vi "LabVIEW Measurement UI - Verify Parameter Matching.vi"(0 "Measurement Client Wrapper in":refnum<class "Measurement Client Wrapper.lvclass">, 11 "error in":errorcluster) -> (4 "Measurement Client Wrapper":refnum<class "Measurement Client Wrapper.lvclass">, 6 "Status":string, 8 "Matching?":bool, 15 "error out":errorcluster)   [LabVIEW 2020, in "Measurement Client Wrapper.lvclass"]
uses:
  Measurement Client Wrapper.lvclass
  Measurement Client Wrapper.lvclass/Measurement Client Wrapper.ctl
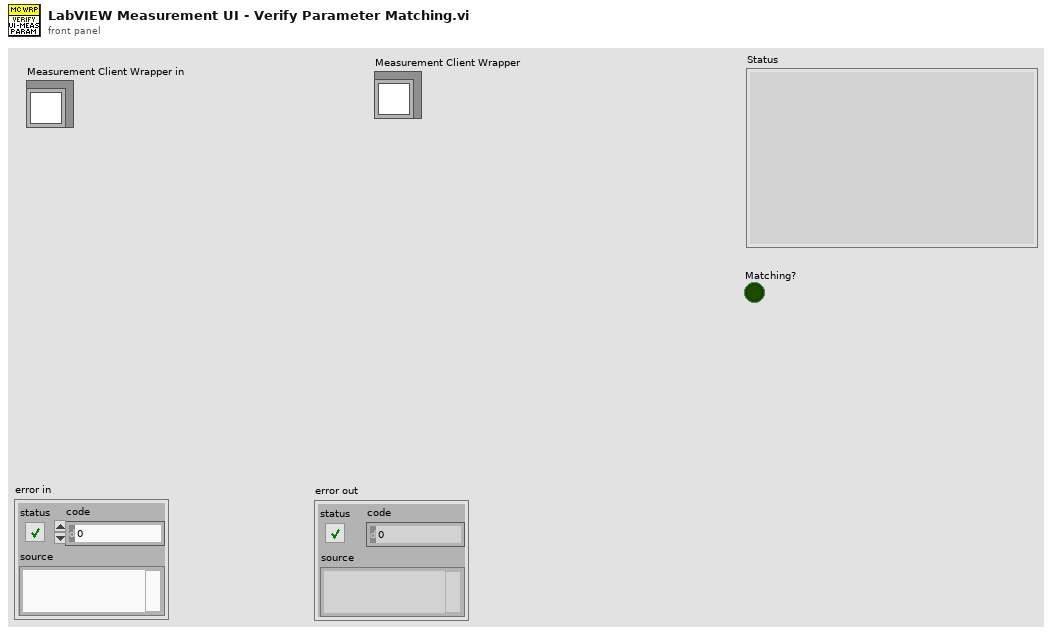
[diagram p1: front panel]
types:
  T1 = typedef "Measurement Client Wrapper.lvclass/MeasurementConfigurationParameters.ctl" = cluster{"protobuf_id":u32, "type":T2, "name":string, "repeated":bool}
  T2 = typedef "Measurement_client-release.lvlib/ni_measurements_v1_Type.ctl" = enum32{"TYPE_UNSPECIFIED", "TYPE_DOUBLE", "TYPE_FLOAT", "TYPE_INT64", "TYPE_UINT64", "TYPE_INT32", "TYPE_FIXED64", "TYPE_FIXED32", "TYPE_BOOL", "TYPE_STRING", "TYPE_GROUP", "TYPE_MESSAGE", "TYPE_BYTES", "TYPE_UINT32", "TYPE_ENUM", "TYPE_SFIXED32", "TYPE_SFIXED64", "TYPE_SINT32", "TYPE_SINT64"}
  T3 = typedef "Measurement Client Wrapper.lvclass/MeasurementOutputParameters.ctl" = cluster{"protobuf_id":u32, "type":T2, "name":string, "repeated":bool}
  T4 = typedef "Measurement Client Wrapper.lvclass/Control UI MetaData.ctl" = cluster{"Name":string, "Parent":string, "LabVIEW DataType":T5, "Measurement DataType":T2, "Value":variant, "1D Array?":bool}
  T5 = typedef "NI_Data Type.lvlib/Data Type.ctl" = enum8{"Invalid Type", "Void", "I8", "I16", "I32", "I64", "U8", "U16", "U32", "U64", "Single Float", "Double Float", "Extended Float", "Single Complex", "Double Complex", "Extended Complex", "Enum U8", "Enum U16", "Enum U32", "Enum U64", "Single Float With Unit", "Double Float With Unit", "Extended Float With Unit", "Single Complex with Unit", "Double Complex with Unit", "Extended Complex with Unit", "Boolean", "String", "Path", "Picture", "Tag", "Array", "Cluster", "Variant", "LV Variant", "Waveform", "Timestamp", "Digital Waveform", "Digital Data", "ExpressData", "Refnum", "External Data", "VI", "Poly VI", "LabVIEW Class Instance", "Fixed Point", "Set Collection", "Map Collection"}
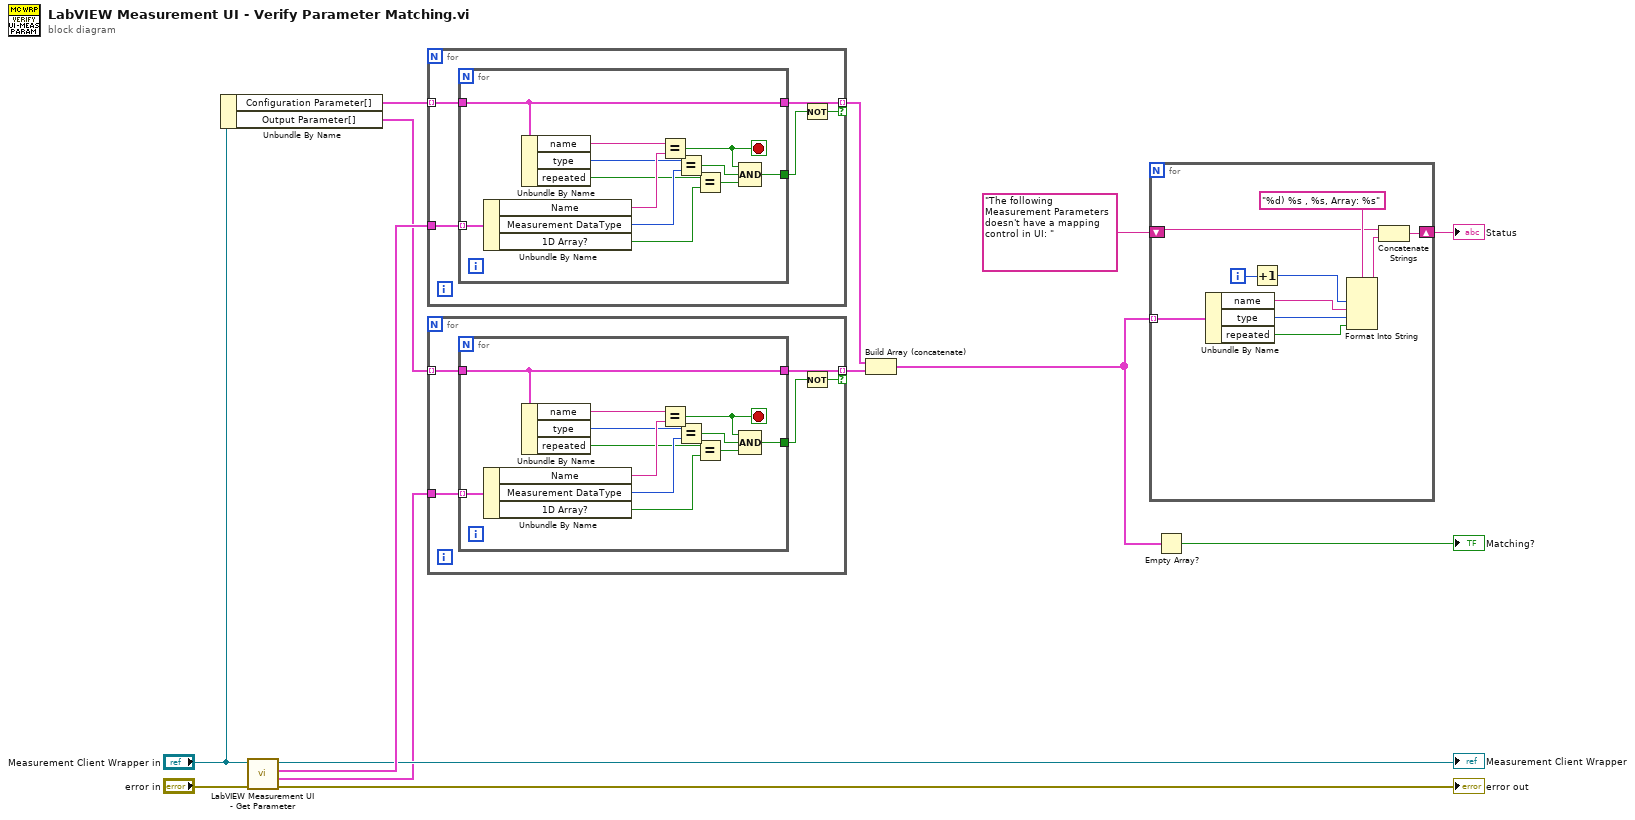
[diagram p0: block diagram]
diagram:
  n1 = Unbundle By Name("Measurement Client Wrapper in") -> ("Configuration Parameter[]"=w9:T1[], "Output Parameter[]"=w3:T3[])
  n2 = call "LabVIEW Measurement UI - Get Parameter.vi"("error in"="error in", "Measurement Client Wrapper in"="Measurement Client Wrapper in") -> ("error out"=→"error out":errorcluster, "UI Indicator Details[]"=w2:T4[], "UI Control Details[]"=w5:T4[], "Measurement Client Wrapper"=→"Measurement Client Wrapper":refnum<class "Measurement Client Wrapper.lvclass">)  [unwired: 6 in]
  n3 = for {
    tunnel: w9 -> [w18] mode=indexing
    tunnel: w5 -> [w19]
    tunnel: [w17] -> w14 mode=indexing if=w15
    n4 = for {
      tunnel: w19 -> [w31] mode=indexing
      tunnel: [w23] -> w16
      tunnel: w18 -> [w24]
      tunnel: [w24] -> w17
      stop <- w28 stop-if-true
      n5 = Unbundle By Name(w31) -> ("Name"=w30:string, "Measurement DataType"=w29:T2, "1D Array?"=w21:bool)
      n6 = Unbundle By Name(w24) -> ("name"=w26:string, "type"=w25:T2, "repeated"=w22:bool)
      n7 = Equal?(x=w26, y=w30) -> (x = y?=w28:bool)
      n8 = Equal?(x=w25, y=w29) -> (x = y?=w27:bool)
      n9 = Equal?(x=w22, y=w21) -> (x = y?=w20:bool)
      n10 = Compound Arithmetic op=AND(w28, w27, w20) -> (w23:bool)
    }
    n11 = Not(x=w16) -> (.not. x?=w15:bool)
  }
  n12 = for {
    tunnel: w3 -> [w35] mode=indexing
    tunnel: w2 -> [w36]
    tunnel: [w34] -> w1 mode=indexing if=w32
    n13 = for {
      tunnel: w36 -> [w48] mode=indexing
      tunnel: [w40] -> w33
      tunnel: w35 -> [w41]
      tunnel: [w41] -> w34
      stop <- w45 stop-if-true
      n14 = Unbundle By Name(w48) -> ("Name"=w47:string, "Measurement DataType"=w46:T2, "1D Array?"=w38:bool)
      n15 = Unbundle By Name(w41) -> ("name"=w43:string, "type"=w42:T2, "repeated"=w39:bool)
      n16 = Equal?(x=w43, y=w47) -> (x = y?=w45:bool)
      n17 = Equal?(x=w42, y=w46) -> (x = y?=w44:bool)
      n18 = Equal?(x=w39, y=w38) -> (x = y?=w37:bool)
      n19 = Compound Arithmetic op=AND(w45, w44, w37) -> (w40:bool)
    }
    n20 = Not(x=w33) -> (.not. x?=w32:bool)
  }
  n21 = Build Array (concatenate)(w14, w1) -> (w11:T3[])
  n22 = for {
    tunnel: w11 -> [w58] mode=indexing
    shift-right: [w52] -> w12
    shift-left: "The following Measurement Parameters doesn't have a mapping control in UI: " ("format string") -> [w51]
    i -> [w54]
    n23 = Unbundle By Name(w58) -> ("name"=w55:string, "type"=w57:T2, "repeated"=w49:bool)
    n24 = Increment(x=w54) -> (x+1=w53:i32)
    n25 = Format Into String(format string="%d) %s , %s, Array: %s", w53, w55, w57, w49) -> (resulting string=w50:string)  [unwired: 2 in, 1 out]
    n26 = Concatenate Strings(w51, w50) -> (w52:string)
  }
  "Status" <- w12
  n27 = Empty Array?(array=w11) -> (empty?=→"Matching?":bool)
